vi "Initialize.vi"(8 "error in (no error)":errorcluster, 9 "Msg Ref":refnum<vi>, 10 "Name":string, 11 "Filter Wheel in":refnum<class "Filter Wheel.lvclass">) -> (0 "error out":errorcluster, 3 "Filter Wheel out":refnum<class "Filter Wheel.lvclass">)   [LabVIEW 2024, in "Filter Wheel.lvclass"]
uses:
  Filter Wheel Object/Filter Wheel.lvclass
  Filter Wheel Object/Filter Wheel.lvclass/Filter Wheel.ctl
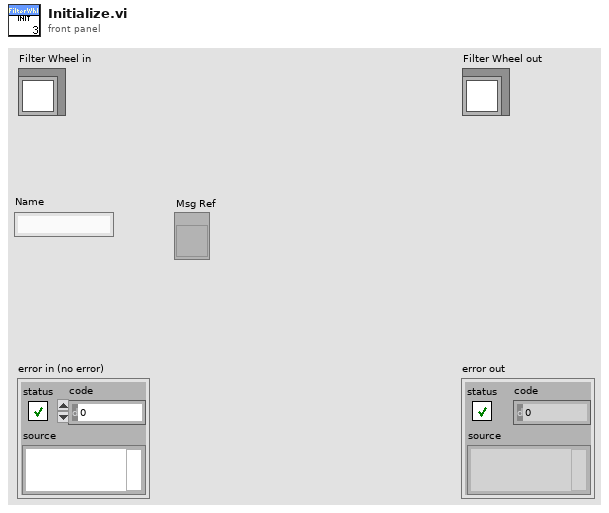
[diagram p1: front panel]
types:
  T1 = typedef "Filter Wheel.lvclass/Filter Wheel configuration.ctl" = cluster{"Num Wheels":i32, "Filters":T2[], "Invalid Combinations":i32[][], "Addr":refnum<visa-resource-name>, "Name":string, "Simulate":bool, "Default Speed":u16, "Homing":T3[]}
  T2 = typedef "Filter Wheel.lvclass/Filter Wheel Details.ctl" = cluster{"Names":string[], "Relative Position":i32[], "Wheel Name":string, "Size":i32}
  T3 = typedef "Filter Wheel Arduino Homing cluster.ctl" = cluster{"Direction":bool, "Speed":i32, "Accel":i32, "Error Cnts":i32, "Homing Delta":i32}
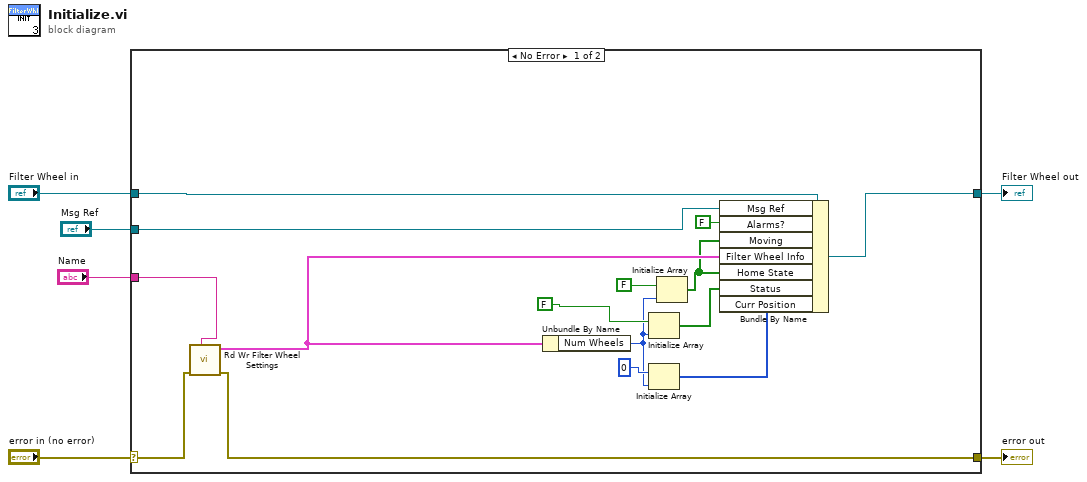
[diagram p0: block diagram]
diagram:
  n1 = case shown="No Error" "error in (no error)" {
    selector: "error in (no error)" -> [w21 w23]
    tunnel: [w20 w23] -> w5
    tunnel: [w15 w22] -> w3
    tunnel: "Filter Wheel in" -> [w13 w22]
    tunnel: "Name" -> [w11 _]
    tunnel: "Msg Ref" -> [w7 _]
    frame No Error {
      n2 = call "Rd Wr Filter Wheel Settings.vi"("Wheel Name"=w11, "error in (no error)"=w21) -> ("error out"=w20:errorcluster, "Filter Wheel Settings"=w16:T1)  [unwired: 8 in]
      n3 = Unbundle By Name(w16) -> ("Num Wheels"=w8:i32)
      n4 = Initialize Array(FALSE, w8) -> (w19:bool[])
      n5 = Initialize Array(0 ("Numeric"), w8) -> (w17:i32[])
      n6 = Initialize Array(FALSE, w8) -> (w10:bool[])
      n7 = Bundle By Name(cluster=w13, "Msg Ref"=w7, "Alarms?"=FALSE, "Moving"=w10, "Filter Wheel Info"=w16, "Home State"=w10, "Status"=w19, "Curr Position"=w17) -> (w15:refnum<class "Filter Wheel.lvclass">)
    }
    frame Error {
    }
  }
  "error out" <- w5
  "Filter Wheel out" <- w3
